vi "Sprache bei den Elementen aendern_IB.vi"(5 "Datei erstellen":bool, 7 "Index (Seite)":i32, 10 "Sprachauswahl":u16, 11 "VI Referenzen":refnum<vi>[](array[refnum])) -> ()   [LabVIEW 2020, in "Sprachverwaltung.lvlib"]
uses:
  Sprachverwaltung.lvlib
  FGV Aktion Tabelle zerlegen.ctl
  Allgemein/allgemeine Sub-VIs.lvlib
  <vilib>/Utility/file.llb/Write Delimited Spreadsheet (string).vi
panel:
  out "KlassenID":u32[](array[numeric])
  # "3 Generic \n4 Decoration \n5 Text \n6 Control \n7 ColorBox \n8 Boolean \n9 RefNum \n10 Variant \n11 Path \n12 ListBox \n13 Table \n14 Array \n15 Picture \n16 ActiveXContainer \n17 Numeric \n18 Digital \n19 NamedNumeric \n20 ColorRamp \n21 Slide \n22 GraphOrChart \n23 WaveformChart \n24 WaveformGraph \n25 IntensityChart \n26 IntensityGraph \n27 String \n28 IOName \n29 ComboBox \n30 Cluster \n31 Panel \n32 Knob \n33 NumWithScale \n34 Ring \n35 Enum \n36 GObject \n37 Plot \n38 Cursor \n39 NumericText \n40 Scale \n41 ColorScale \n42 GraphScale \n43 ColorGraphScale \n44 TypedRefNum \n45 OldKnobScale \n46 MCListbox \n47 MeasureData \n48 BVTag \n49 DAQName \n50 VISAName \n51 IVIName \n52 SlideScale \n54 Page \n55 TabControl \n56 ConPane"
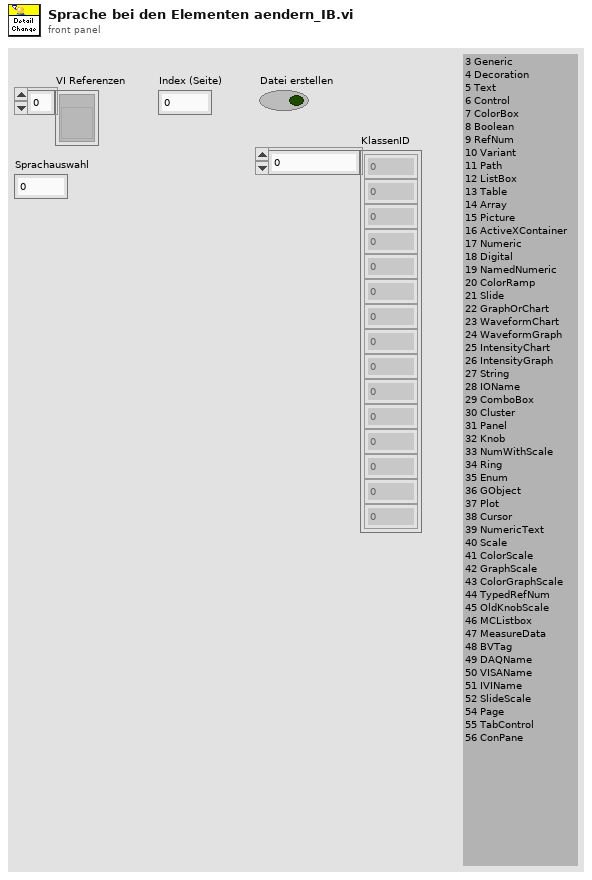
[diagram p1: front panel]
types:
  T1 = typedef "Sprachverwaltung.lvlib/FGV Aktion Tabelle zerlegen.ctl" = enum16{"laden", "vereinzeln", "speichern"}
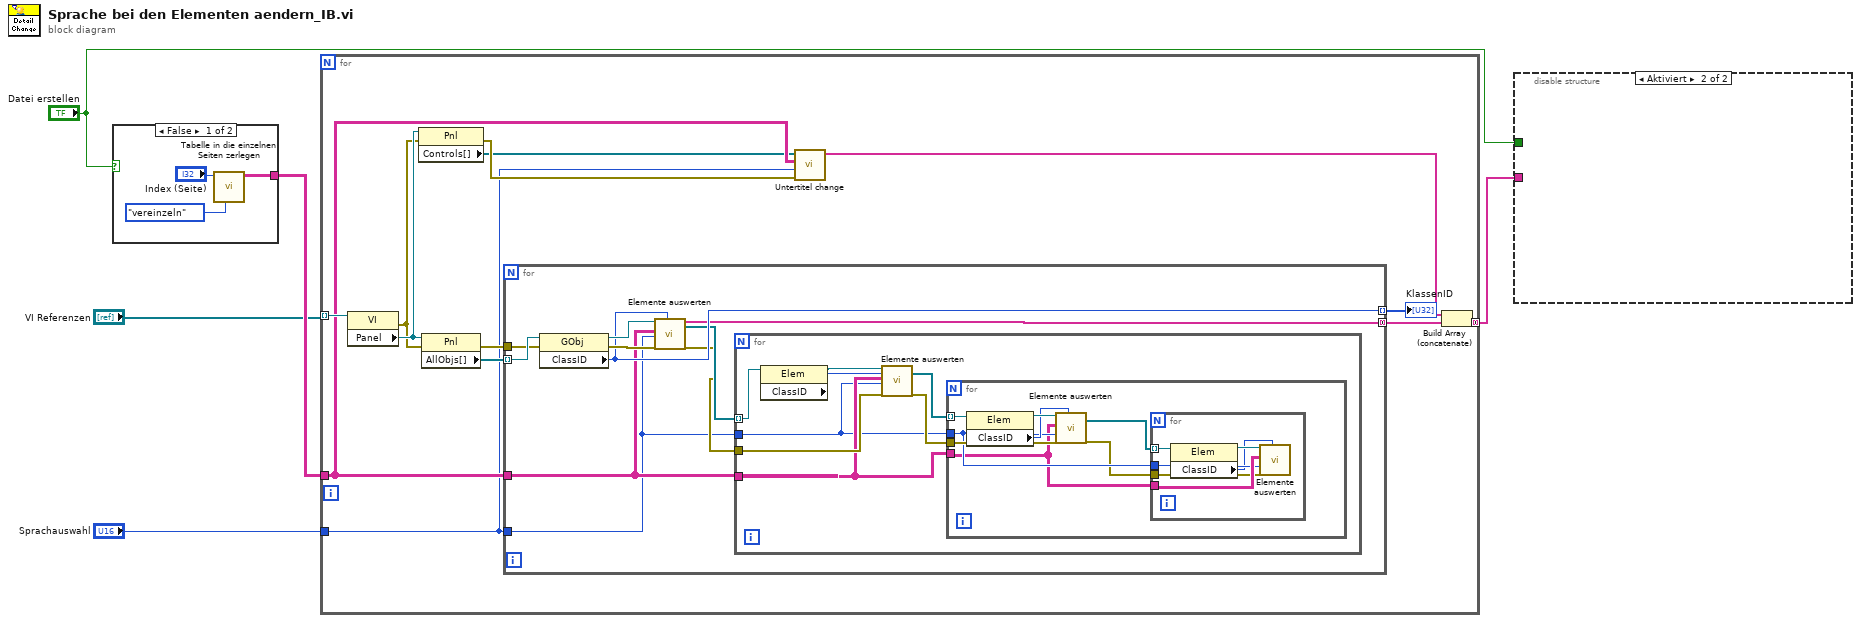
[diagram p0: block diagram]
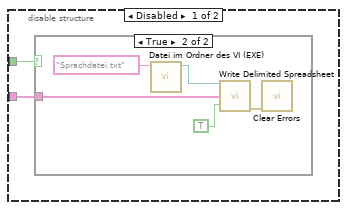
[diagram p2: hidden frame]
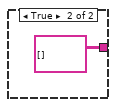
[diagram p4: hidden frame]
diagram:
  n1 = case shown="False" "Datei erstellen" {
    tunnel: [w8 string[][] [] ("all rows")] -> w5
    frame False {
      n2 = call "Tabelle in die einzelnen Seiten zerlegen.vi"("Aktion"=FGV_Aktion_Tabelle_zerlegen."vereinzeln", "Index (Seite)"="Index (Seite)") -> ("Sprachliste"=w8:string[][])  [unwired: 7 in, 2 out]
    }
    frame True {
    }
  }
  n3 = for {
    tunnel: "VI Referenzen" -> [w19] mode=indexing
    tunnel: w5 -> [w17]
    tunnel: "Sprachauswahl" -> [w13]
    tunnel: [w11] -> w2 mode=concatenating
    n4 = property class="VI"(reference=w19) -> (error out=w16:errorcluster, "Panel"=w18:refnum<vi>)  [unwired: 1 in, 1 out]
    n5 = property class="Pnl"(reference=w18, error in=w16) -> (error out=w15:errorcluster, "Controls[]"=w14:refnum<vi>[])  [unwired: 1 out]
    n6 = property class="Pnl"(reference=w18, error in=w16) -> (error out=w20:errorcluster, "AllObjs[]"=w22:refnum<vi>[])  [unwired: 1 out]
    n7 = for {
      tunnel: w22 -> [w32] mode=indexing
      tunnel: w17 -> [w24]
      tunnel: w13 -> [w23]
      tunnel: [w29] -> w21 mode=indexing
      tunnel: w20 -> [w28]
      tunnel: [w27] -> w12 mode=concatenating
      n8 = property class="GObj"(reference=w32, error in=w28) -> (reference out=w31:refnum<vi>, error out=w30:errorcluster, "ClassID"=w29:u32)
      n9 = call "Elemente auswerten.vi"("GObject (Eingang)"=w31, "all rows"=w24, "Sprachauswahl"=w23, "Fehler (Eingang, kein Fehler)"=w30, "ClassID"=w29) -> ("Strings [4]"=w27:string[], "Cluster Elemente[]"=w26:refnum<vi>[], "error out"=w25:errorcluster)  [unwired: 12 in]
      n10 = for {
        tunnel: w26 -> [w39] mode=indexing
        tunnel: w24 -> [w36]
        tunnel: w23 -> [w34]
        tunnel: w25 -> [w40]
        n11 = property class="Elem"(reference=w39) -> (reference out=w38:refnum<vi>, "ClassID"=w37:u32)  [unwired: 1 in, 1 out]
        n12 = call "Elemente auswerten.vi"("GObject (Eingang)"=w38, "all rows"=w36, "Sprachauswahl"=w34, "Fehler (Eingang, kein Fehler)"=w40, "ClassID"=w37) -> ("Cluster Elemente[]"=w33:refnum<vi>[], "error out"=w35:errorcluster)  [unwired: 12 in, 1 out]
        n13 = for {
          tunnel: w36 -> [w41]
          tunnel: w35 -> [w48]
          tunnel: w34 -> [w43]
          tunnel: w33 -> [w47] mode=indexing
          n14 = property class="Elem"(reference=w47) -> (reference out=w46:refnum<vi>, "ClassID"=w45:u32)  [unwired: 1 in, 1 out]
          n15 = call "Elemente auswerten.vi"("GObject (Eingang)"=w46, "all rows"=w41, "Sprachauswahl"=w43, "Fehler (Eingang, kein Fehler)"=w48, "ClassID"=w45) -> ("Cluster Elemente[]"=w44:refnum<vi>[], "error out"=w42:errorcluster)  [unwired: 12 in, 1 out]
          n16 = for {
            tunnel: w41 -> [w54]
            tunnel: w42 -> [w53]
            tunnel: w43 -> [w52]
            tunnel: w44 -> [w51] mode=indexing
            n17 = property class="Elem"(reference=w51) -> (reference out=w50:refnum<vi>, "ClassID"=w49:u32)  [unwired: 1 in, 1 out]
            n18 = call "Elemente auswerten.vi"("GObject (Eingang)"=w50, "all rows"=w54, "Sprachauswahl"=w52, "Fehler (Eingang, kein Fehler)"=w53, "ClassID"=w49) -> ()  [unwired: 12 in, 3 out]
          }
        }
      }
    }
    "KlassenID" <- w21
    n19 = call "Untertitel change.vi"("Fehler (Eingang, kein Fehler)"=w15, "Sprachauswahl"=w13, "Sprachdatei"=w17, "Controls[]"=w14) -> ("Untertiteln"=w10:string[])  [unwired: 6 in, 1 out]
    n20 = Build Array (concatenate)(w10, w12) -> (w11:string[])
  }
  n21 = disable-structure shown="Aktiviert" {
    disable-tunnel: w2 -> [w56 _]
    disable-tunnel: "Datei erstellen" -> [w55 _]
    frame Disabled {
      n22 = case shown="True" w55 {
        tunnel: w56 -> [_ w59]
        frame False {
        }
        frame True {
          n23 = call "Datei im Ordner des VI (EXE).vi"("Dateiname"="Sprachdatei.txt") -> ("Dateipfad im Ordner des Haupt-VIs"=w61:path)  [unwired: 8 in, 2 out]
          n24 = call-poly <vilib>:"Write Delimited Spreadsheet.vi"("file path (dialog if empty)"=w61, "1D data"=w59, "transpose? (no:F)"=TRUE ("transpose? (F)")) -> ("error out"=w58:errorcluster)  [unwired: 11 in, 1 out]
          n25 = call <vilib>:"Clear Errors.vi"("error in (no error)"=w58) -> ()  [unwired: 5 in, 2 out]
        }
      }
    }
    frame Enabled {
    }
  }
